vi "GRAFICOS.vi"() -> ()   [LabVIEW 2020]
panel:
  in  "stop":bool
  out "Waveform Chart":dbl(graph)
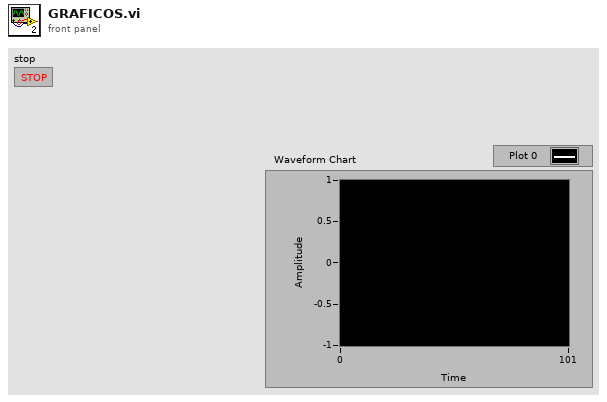
[diagram p1: front panel]
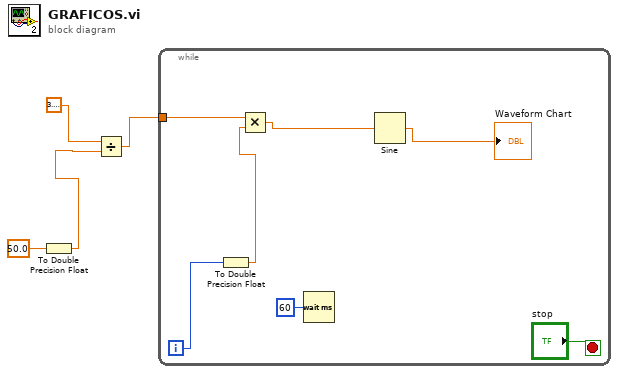
[diagram p0: block diagram]
diagram:
  n1 = To Double Precision Float(number=50.0) -> (double precision float=w2:dbl)
  n2 = Divide(x=3.141592653589793, y=w2) -> (x/y=w3:dbl)
  n3 = while {
    tunnel: w3 -> [w9]
    i -> [w8]
    stop <- "stop" stop-if-true
    n4 = To Double Precision Float(number=w8) -> (double precision float=w7:dbl)
    n5 = Multiply(x=w9, y=w7) -> (x*y=w6:dbl)
    n6 = Wait (ms)(milliseconds to wait=u32 60) -> ()  [unwired: 1 out]
    n7 = Sine(x=w6) -> (sin(x)=→"Waveform Chart":dbl)
  }
